vi "Create Dictionary from File.vi"(8 "error in":errorcluster, 11 "reference in":refnum<class "Electronic Datasheet.lvclass">) -> (0 "error out":errorcluster, 3 "reference out":refnum<class "Electronic Datasheet.lvclass">)   [LabVIEW 2020, in "Electronic Datasheet.lvlib" / "Electronic Datasheet.lvclass"]
uses:
  Electronic Datasheet.lvclass
  Core/Object Dictionary/Dictionary.lvclass
  Electronic Datasheet.lvclass/Electronic Datasheet.ctl
  <vilib>/Utility/config.llb/NI_LVConfig.lvlib
  Core/OD Section/Section.lvclass
  <vilib>/Utility/config.llb/Read Key (String).vi
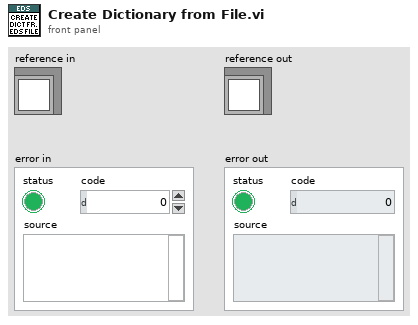
[diagram p1: front panel]
types:
  T1 = typedef "Electronic Datasheet.lvlib/Electronic Datasheet.lvclass/ObjectAttributes.ctl" = cluster{"EDS File Path":path, "Object Dict":refnum<class "Dictionary.lvclass">, "Sorted Object Dict":refnum<class "Sorted Object Dictionary.lvclass">, "Device Info":refnum<class "Device Info.lvclass">, "File Info":refnum<class "File Info.lvclass">}
  T2 = typedef "NI_LVConfig.lvlib/Config Data RefNum.ctl" = refnum<k1>
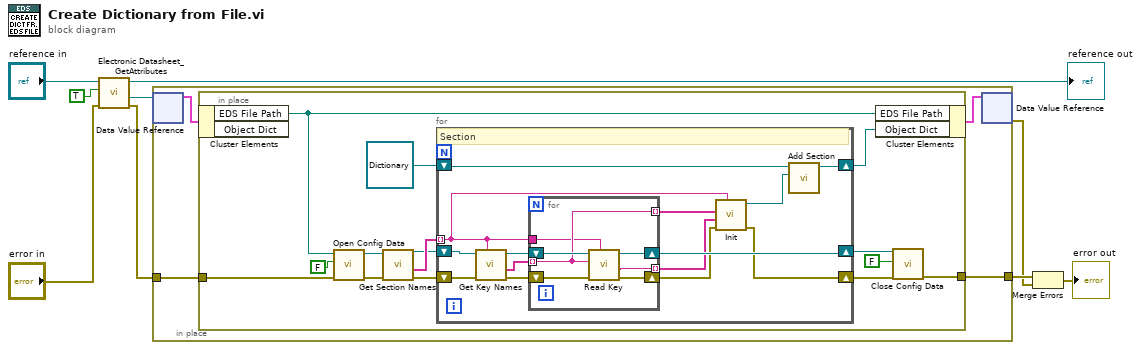
[diagram p0: block diagram]
diagram:
  n1 = call "Electronic Datasheet_GetAttributes.vi"("Error In"="error in", "OnlyGetDvrReference(False)"=TRUE, "reference in"="reference in") -> ("Error Out"=w1:errorcluster, "DataRef"=w5:refnum<data-value>, "reference out"=→"reference out":refnum<class "Electronic Datasheet.lvclass">)  [unwired: 5 in, 1 out]
  n2 = in-place {
    in-place-border: [w13] -> w9
    in-place-border: w1 -> [w10]
    n3 = in-place-dvr #1(w5) -> (w12:T1)  [unwired: 1 out]
    n4 = in-place {
      in-place-border: [w27] -> w13
      in-place-border: w10 -> [w14]
      n5 = in-place-cluster #2(w12) -> ("EDS File Path"=w16:path)  [unwired: 1 out]
      n6 = call <vilib>:"Open Config Data.vi"("error in (no error)"=w14, "create file if necessary (T)"=FALSE, "configuration file path"=w16) -> ("error out"=w17:errorcluster, "refnum"=w18:T2)  [unwired: 6 in, 1 out]
      n7 = call <vilib>:"Get Section Names.vi"("error in (no error)"=w17, "refnum"=w18) -> ("error out"=w20:errorcluster, "section names"=w25:string[], "refnum out"=w21:T2)  [unwired: 7 in]
      n8 = for {
        tunnel: w25 -> [w33] mode=indexing
        shift-right: [w29] -> w22
        shift-left: w20 -> [w41]
        shift-right: [w37] -> w23
        shift-left: w21 -> [w40]
        shift-right: [w35] -> w15
        shift-left: refnum<class "Dictionary.lvclass"> refnum ("Object Dictionary") -> [w34]
        # "Section"
        n9 = call <vilib>:"Get Key Names.vi"("section"=w33, "error in (no error)"=w41, "refnum"=w40) -> ("error out"=w39:errorcluster, "key names"=w36:string[], "refnum out"=w38:T2)  [unwired: 5 in, 1 out]
        n10 = for {
          shift-right: [w44] -> w30
          shift-left: w39 -> [w48]
          tunnel: w36 -> [w43] mode=indexing
          shift-right: [w46] -> w37
          shift-left: w38 -> [w47]
          tunnel: [w45] -> w31 mode=indexing
          tunnel: [w43] -> w32 mode=indexing
          tunnel: w33 -> [w42]
          n11 = call-poly <vilib>:"Read Key.vi"("section"=w42, "error in (no error)"=w48, "key"=w43, "refnum"=w47) -> ("error out"=w44:errorcluster, "value"=w45:string, "refnum out"=w46:T2)  [unwired: 4 in, 1 out]
        }
        n12 = call "Init.vi"("Name"=w33, "error in"=w30, "Values"=w31, "Keynames"=w32) -> ("error out"=w29:errorcluster, "Section out"=w28:refnum<class "Section.lvclass">)  [unwired: 6 in]
        n13 = call "Add Section.vi"("Section"=w28, "Dictionary in"=w34) -> ("Dictionary out"=w35:refnum<class "Dictionary.lvclass">)  [unwired: 9 in]
      }
      n14 = in-place-cluster #2("EDS File Path"=w16, "Object Dict"=w15) -> (w11:T1)
      n15 = call <vilib>:"Close Config Data.vi"("error in (no error)"=w22, "write file if changed (T)"=FALSE, "refnum"=w23) -> ("error out"=w27:errorcluster)  [unwired: 7 in, 1 out]
    }
    n16 = in-place-dvr #1(w11) -> (w2:errorcluster)  [unwired: 1 out]
  }
  n17 = Merge Errors(w9, w2) -> (→"error out":errorcluster)
